vi "AIT 664 - Load Database.vi"(8 "error in (no error)":errorcluster, 11 "Node Ptr":u64 format="%.0x") -> (0 "error out":errorcluster)   [LabVIEW 2015, in "AIT 664 Custom Device.lvlib"]
doc: "Load Simulyzer file, populate device tree, and read in parms file if it exists."
uses:
  AIT 664 Custom Device.lvlib
  <vilib>/NI Veristand/Custom Device API/Custom Device Item Ref.ctl
  <vilib>/NI Veristand/Custom Device API/Set Item Property (Path).vi
  <vilib>/NI Veristand/Custom Device API/Set Item Property (String).vi
  <vilib>/NI Veristand/Custom Device API/Get Item Property (Path).vi
  Controls and Global/Global.vi
  <vilib>/NI Veristand/Custom Device API/Custom Device API.lvlib
  <vilib>/NI Veristand/Custom Device Tools/Custom Device Utility Library/Custom Device Utility Library.lvlib
panel:
  out "Item Ref out 2":T1=18446744073709551615 format="%.0x"
  out "selected path 2":path
  out "Item Ref out":T1=18446744073709551615 format="%.0x"
  out "selected path":path
  out "Node Ptr dup":u64
  out "empty path":bool
  out "Win File Path":string
  in  "Tag":string
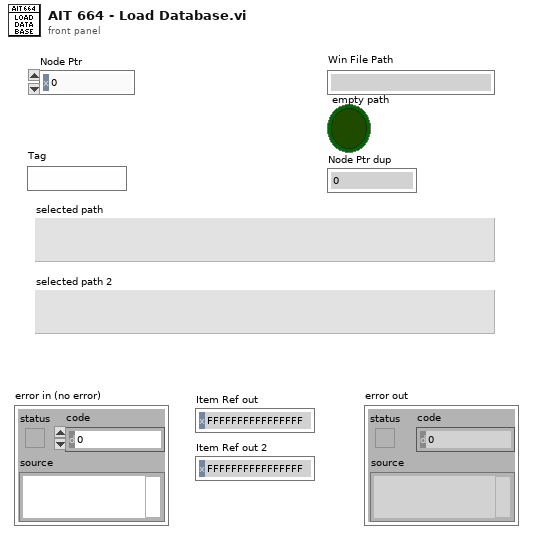
[diagram p1: front panel]
types:
  T1 = typedef "Custom Device API.lvlib/Custom Device Item Ref.ctl" = u64
  T2 = enum32{"Invalid", "Standard", "Closed", "Hidden", "Minimized", "Maximized"}
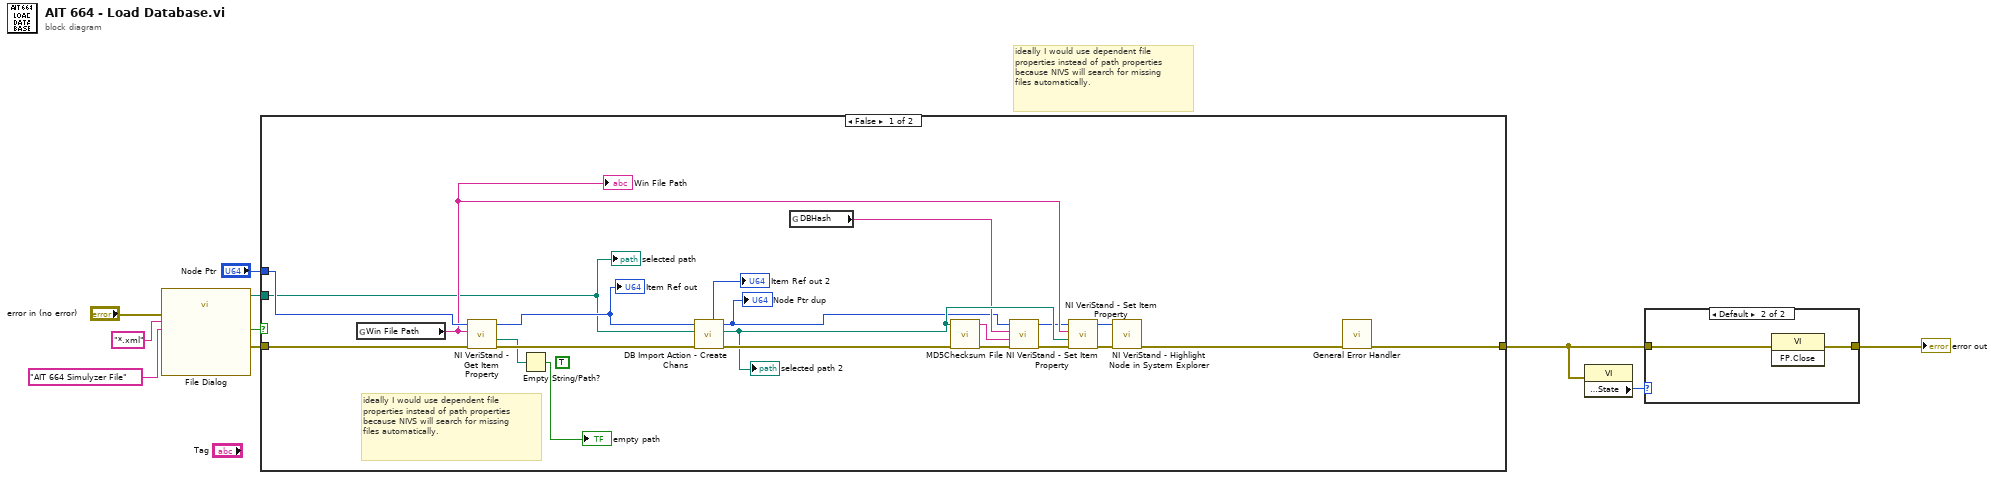
[diagram p0: block diagram]
diagram:
  # "ideally I would use dependent file properties instead of path properties because NIVS will search for missing files automatically."
  n1 = call "File Dialog"("error in"="error in (no error)", "pattern (all files)"="*.xml", "pattern label"="AIT 664 Simulyzer File") -> ("selected path"=w5:path, "cancelled"=w8:bool, "error out"=w7:errorcluster)  [unwired: 9 in, 1 out]
  n2 = case shown="False" w8 {
    tunnel: [w18 w32] -> w3
    tunnel: w7 -> [w28 w32]
    tunnel: "Node Ptr" -> [w27 _]
    tunnel: w5 -> [w22 _]
    frame False {
      (unwired) TRUE
      # "ideally I would use dependent file properties instead of path properties because NIVS will search for missing files automatically."
      n3 = global read "Global.vi" "Win File Path"() -> (w24:string)
      "Win File Path" <- w24
      n4 = call-poly <vilib>:"NI VeriStand - Get Item Property.vi"("error in (no error)"=w28, "Property Name"=w24, "Item Ref in"=w27) -> ("error out"=w25:errorcluster, "Value"=w21:path, "Item Ref out"=w26:T1)  [unwired: 5 in, 1 out]
      "Item Ref out" <- w26
      n5 = Empty String/Path?(string/path=w21) -> (empty?=→"empty path":bool)
      n6 = call "DB Import Action - Create Chans.vi"("error in (no error)"=w25, "selected path"=w22, "Node Ptr"=w26) -> ("error out"=w31:errorcluster, "selected path out"=w30:path, "Node Ptr dup"=w20:u64, "Item Ref"=→"Item Ref out 2":T1)  [unwired: 5 in]
      "Node Ptr dup" <- w20
      "selected path 2" <- w30
      n7 = global read "Global.vi" "DBHash"() -> (w29:string)
      n8 = call <vilib>:"MD5Checksum File.vi"("error in (no error)"=w31, "Path"=w30) -> ("error out"=w12:errorcluster, "MD5 message-digest"=w11:string)  [unwired: 8 in]
      n9 = call-poly <vilib>:"NI VeriStand - Set Item Property.vi"("error in (no error)"=w12, "Value"=w11, "Property Name"=w29, "Item Ref in"=w20) -> ("error out"=w13:errorcluster, "Item Ref out"=w14:T1)  [unwired: 5 in, 1 out]
      n10 = call-poly <vilib>:"NI VeriStand - Set Item Property.vi"("error in (no error)"=w13, "Value"=w30, "Property Name"=w24, "Item Ref in"=w14) -> ("error out"=w16:errorcluster, "Item Ref out"=w15:T1)  [unwired: 5 in, 1 out]
      n11 = call <vilib>:"NI VeriStand - Highlight Node in System Explorer.vi"("error in (no error)"=w16, "Item Ref in"=w15) -> ("error out"=w19:errorcluster)  [unwired: 8 in, 1 out]
      n12 = call <vilib>:"General Error Handler.vi"("error in (no error)"=w19) -> ("error out"=w18:errorcluster)  [unwired: 10 in, 4 out]
      "selected path" <- w22
    }
    frame True {
    }
  }
  n13 = property class="VI"(error in=w3) -> ("Front Panel Window:State"=w1:T2)  [unwired: 1 in, 2 out]
  n14 = case shown="Default" w1 {
    tunnel: [w33 w35] -> w2
    tunnel: w3 -> [w33 w34]
    frame "Closed" {
    }
    frame Default {
      n15 = invoke class="VI" method="FP.Close"(error in=w34) -> (error out=w35:errorcluster)  [unwired: 2 in, 2 out]
    }
  }
  "error out" <- w2
